vi "IR sensor.vi"(10 "IR climber clear":T1, 11 "IR sensor disc":T1) -> ()   [LabVIEW 2012]
uses:
  <vilib>/Rock Robotics/SystemInterfaces/AnalogTrigger/FPGA_AnalogTriggerDevRef.ctl
  <vilib>/Rock Robotics/SystemInterfaces/AnalogTrigger/FPGA_AnalogTriggerIndex.ctl
  Robot Global Data.vi
panel:
  in  "IR climber clear":T1
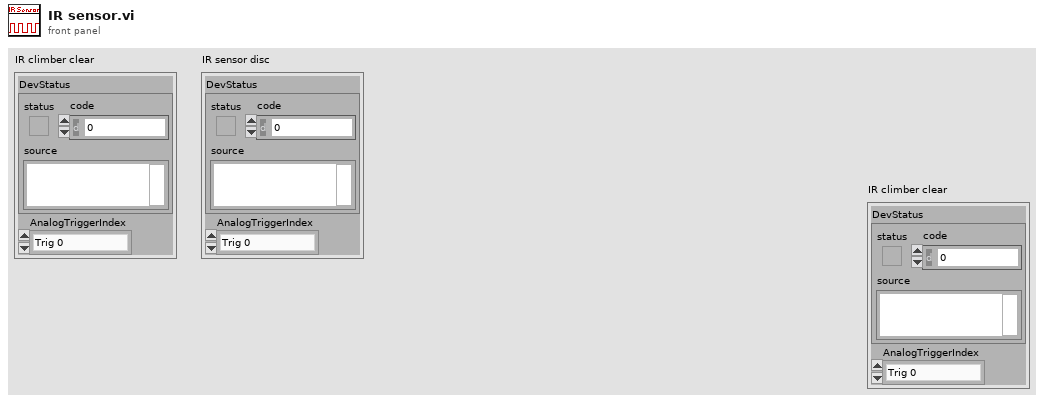
[diagram p1: front panel]
types:
  T1 = typedef "FPGA_AnalogTriggerDevRef.ctl" = cluster{"DevStatus":errorcluster, "AnalogTriggerIndex":T2}
  T2 = typedef "FPGA_AnalogTriggerIndex.ctl" = enum8{"Trig 0", "Trig 1", "Trig 2", "Trig 3", "Trig 4", "Trig 5", "Trig 6", "Trig 7", "Invalid"}
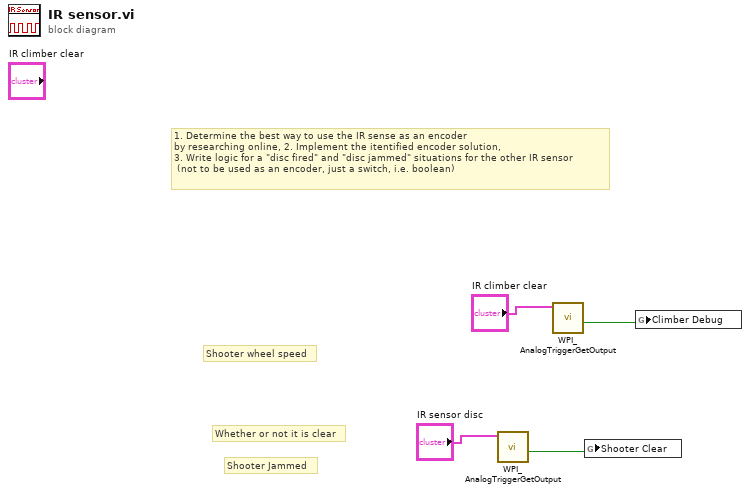
[diagram p0: block diagram]
diagram:
  # "Whether or not it is clear"
  # "Shooter wheel speed"
  # "1. Determine the best way to use the IR sense as an encoder \nby researching online, 2. Implement the itentified encoder solution, \n3. Write logic for a \"disc fired\" and \"disc jammed\" situations for the other IR sensor\n (not to be used as an encoder, just a switch, i.e. boolean)"
  # "Shooter Jammed"
  n1 = call <vilib>:"WPI_AnalogTriggerGetOutput.vi"("AnalogTriggerDevRef"="IR sensor disc") -> ("Trigger State"=w3:bool)  [unwired: 7 in, 3 out]
  n2 = call <vilib>:"WPI_AnalogTriggerGetOutput.vi"("AnalogTriggerDevRef"="IR climber clear") -> ("Trigger State"=w1:bool)  [unwired: 7 in, 3 out]
  n3 = global write "Robot Global Data.vi" "Shooter Clear"(w3) -> ()
  n4 = global write "Robot Global Data.vi" "Climber Debug"(w1) -> ()
